vi "Rotate Active Pixels.vi"(8 "error in (no error)":errorcluster, 10 "Rotate":bool, 11 "Game Engine in":refnum<class "Game Engine.lvclass">) -> (0 "error out":errorcluster, 3 "Game Engine out":refnum<class "Game Engine.lvclass">)   [LabVIEW 2017, in "Game Engine.lvlib" / "Game Engine.lvclass"]
uses:
  Game Engine.lvclass
  Game Engine.lvclass/Game Engine.ctl
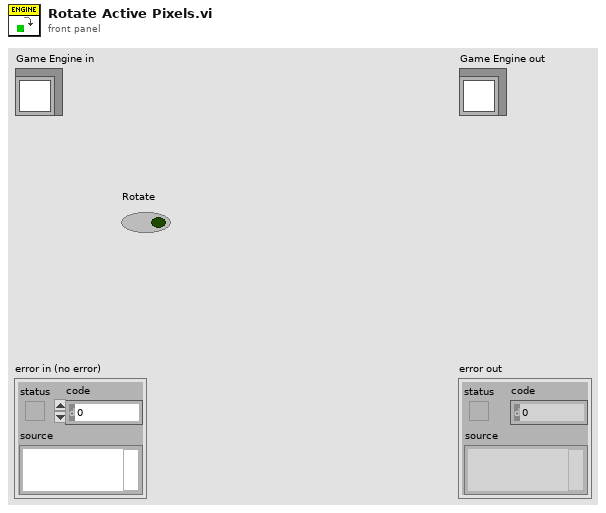
[diagram p1: front panel]
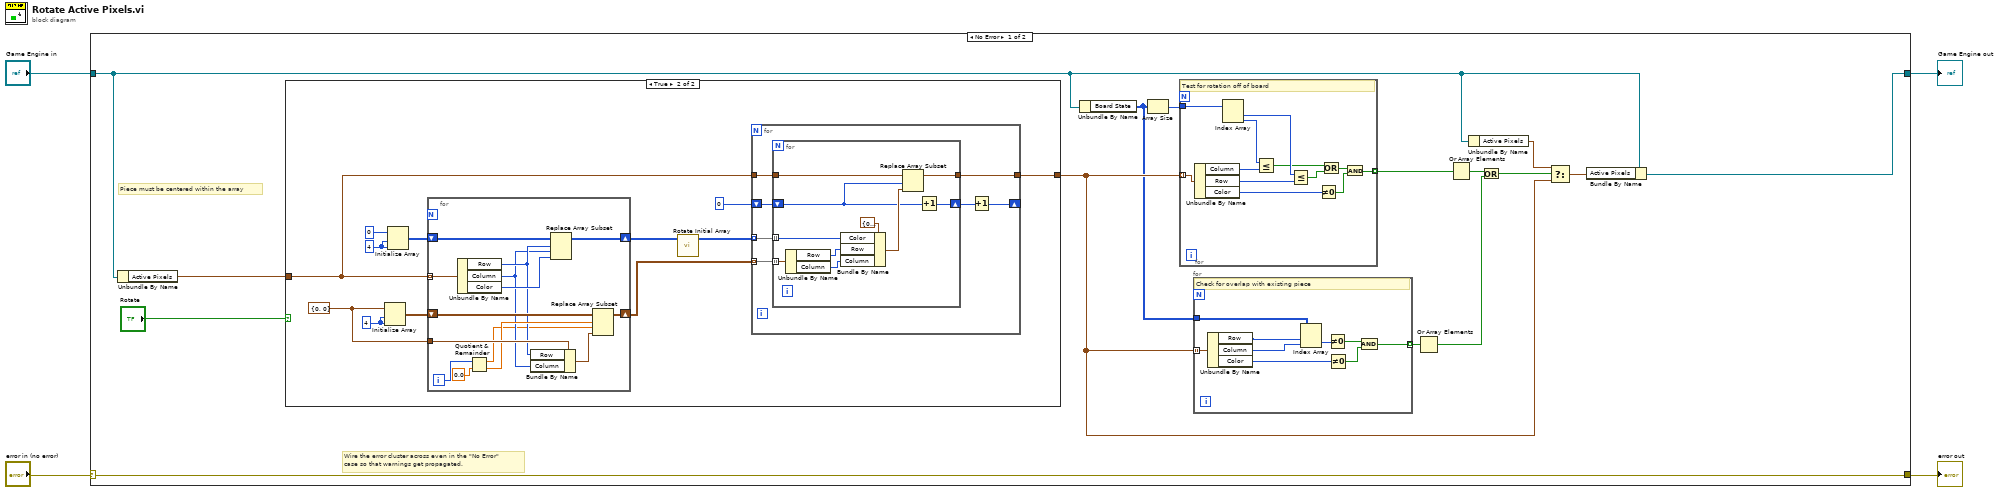
[diagram p0: block diagram]
diagram:
  n1 = case shown="No Error" "error in (no error)" {
    selector: "error in (no error)" -> [w19 w86]
    tunnel: [w19 w86] -> w3
    tunnel: [w17 w85] -> w1
    tunnel: "Game Engine in" -> [w11 w85]
    frame No Error {
      # "Piece must be centered within the array"
      # "Wire the error cluster across even in the \"No Error\"\ncase so that warnings get propagated."
      n2 = Unbundle By Name(w11) -> ("Active Pixels"=w18:cluster{"Column":u8, "Row":u8, "Color":u32}[])
      n3 = case shown="True" "Rotate" {
        tunnel: w18 -> [w41 w48]
        tunnel: [w41 w47] -> w9
        frame False {
        }
        frame True {
          w46 = 4 ("dimension size")
          w44 = cluster{"Row":u8, "Column":u8} {"Row"=0, "Column"=0}
          w52 = 4 ("dimension size")
          n4 = Initialize Array(w44, w46, w46) -> (w45:cluster{"Row":u8, "Column":u8}[][])
          n5 = Initialize Array(u32 0, w52, w52) -> (w51:u32[][])
          n6 = for {
            tunnel: w48 -> [w84] mode=indexing
            shift-right: [w81] -> w50
            shift-left: w51 -> [w83]
            shift-right: [w79] -> w43
            shift-left: w45 -> [w80]
            tunnel: w44 -> [w78]
            i -> [w77]
            n7 = Unbundle By Name(w84) -> ("Row"=w74:u8, "Column"=w73:u8, "Color"=w82:u32)
            n8 = Quotient & Remainder(x=w77, y=0.0) -> (x-y*floor(x/y)=w72:dbl, floor(x/y)=w75:dbl)
            n9 = Bundle By Name(cluster=w78, "Row"=w74, "Column"=w73) -> (w71:cluster{"Row":u8, "Column":u8})
            n10 = Replace Array Subset(array=w83, new element=w82, index (row)=w74, index (col)=w73) -> (w81:u32[][])
            n11 = Replace Array Subset(array=w80, new element=w71, index (row)=w75, index (col)=w72) -> (w79:cluster{"Row":u8, "Column":u8}[][])
          }
          n12 = call "Rotate Initial Array.vi"("Array in"=w50) -> ("Array out"=w49:u32[][])  [unwired: 10 in]
          n13 = for {
            tunnel: w49 -> [w60] mode=indexing
            tunnel: w48 -> [w59]
            tunnel: [w58] -> w47
            tunnel: w43 -> [w57] mode=indexing
            shift-right: [w54] -> _
            shift-left: 0 ("index") -> [w56]
            n14 = for {
              tunnel: w60 -> [w70] mode=indexing
              tunnel: w59 -> [w69]
              tunnel: [w66] -> w58
              tunnel: w57 -> [w65] mode=indexing
              shift-right: [w61] -> w55
              shift-left: w56 -> [w62]
              n15 = Unbundle By Name(w65) -> ("Row"=w64:u8, "Column"=w63:u8)
              n16 = Bundle By Name(cluster=cluster{"Column":u8, "Row":u8, "Color":u32} {"Column"=0, "Row"=0, "Color"=0} ("Active Piece Pixels"), "Color"=w70, "Row"=w64, "Column"=w63) -> (w68:cluster{"Column":u8, "Row":u8, "Color":u32})
              n17 = Replace Array Subset(array=w69, new element=w68, index=w62) -> (w66:cluster{"Column":u8, "Row":u8, "Color":u32}[])
              n18 = Increment(x=w62) -> (x+1=w61:i32)
            }
            n19 = Increment(x=w55) -> (x+1=w54:i32)
          }
        }
      }
      n20 = Unbundle By Name(w11) -> ("Board State"=w8:u32[][])
      n21 = Array Size(array=w8) -> (size(s)=w15:i32[])
      n22 = for {
        tunnel: w9 -> [w40] mode=indexing
        tunnel: w15 -> [w39]
        tunnel: [w29] -> w14 mode=indexing
        # "Test for rotation off of board"
        n23 = Unbundle By Name(w40) -> ("Column"=w38:u8, "Row"=w36:u8, "Color"=w32:u32)
        n24 = Index Array(array=w39) -> (element #1=w35:i32, element #2=w37:i32)  [unwired: 2 in]
        n25 = Less Or Equal?(x=w37, y=w38) -> (x <= y?=w33:bool)
        n26 = Less Or Equal?(x=w35, y=w36) -> (x <= y?=w34:bool)
        n27 = Not Equal To 0?(x=w32) -> (x != 0?=w31:bool)
        n28 = Or(x=w33, y=w34) -> (x .or. y?=w30:bool)
        n29 = And(x=w30, y=w31) -> (x .and. y?=w29:bool)
      }
      n30 = for {
        tunnel: w9 -> [w28] mode=indexing
        tunnel: w8 -> [w27]
        tunnel: [w20] -> w10 mode=indexing
        # "Check for overlap with existing piece"
        n31 = Unbundle By Name(w28) -> ("Row"=w24:u8, "Column"=w26:u8, "Color"=w23:u32)
        n32 = Index Array(array=w27, index (row)=w24, index (col)=w26) -> (element=w25:u32)
        n33 = Not Equal To 0?(x=w25) -> (x != 0?=w22:bool)
        n34 = Not Equal To 0?(x=w23) -> (x != 0?=w21:bool)
        n35 = And(x=w22, y=w21) -> (x .and. y?=w20:bool)
      }
      n36 = Or Array Elements(Boolean array=w10) -> (logical OR=w6:bool)
      n37 = Or Array Elements(Boolean array=w14) -> (logical OR=w7:bool)
      n38 = Unbundle By Name(w11) -> ("Active Pixels"=w12:cluster{"Column":u8, "Row":u8, "Color":u32}[])
      n39 = Or(x=w7, y=w6) -> (x .or. y?=w5:bool)
      n40 = Select(t=w12, s=w5, f=w9) -> (s? t:f=w13:cluster{"Column":u8, "Row":u8, "Color":u32}[])
      n41 = Bundle By Name(cluster=w11, "Active Pixels"=w13) -> (w17:refnum<class "Game Engine.lvclass">)
    }
    frame Error {
    }
  }
  "error out" <- w3
  "Game Engine out" <- w1
